vi "test.vi"() -> ()   [LabVIEW 2023]
uses:
  PXI-5441_class/DC Config_class/DC Config.lvclass
  PXI-5441_class/PXI-5441.lvclass
  D:/git/HAL/PXI-5441_class/PXI-5441.lvclass
  D:/git/HAL/FGEN_class/FGEN.lvclass
  D:/git/HAL/Hardware_class/Hardware.lvclass
  D:/git/HAL/PXI-5441_class/DC Config_class/DC Config.lvclass
  D:/git/HAL/PXI-5441_class/IConfigure_interface/IConfigure.lvclass
panel:
  in  "Resource Name":refnum<k15>
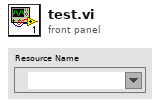
[diagram p1: front panel]
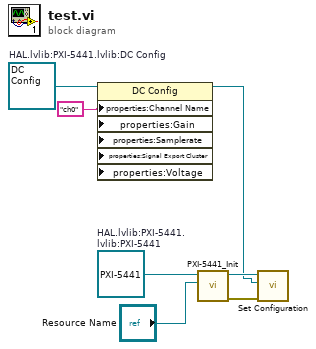
[diagram p0: block diagram]
diagram:
  w7 = refnum<class "PXI-5441.lvclass"> refnum  # HAL.lvlib:PXI-5441.lvlib:PXI-5441
  w3 = refnum<class "DC Config.lvclass"> refnum  # HAL.lvlib:PXI-5441.lvlib:DC Config
  n1 = property class="DC Config" props=["properties:Channel Name", "properties:Gain", "properties:Samplerate", "properties:Signal Export Cluster", "properties:Voltage"](reference=w3, "properties:Channel Name"="ch0" ("Channel Name")) -> (reference out=w2:refnum<class "DC Config.lvclass">)  [unwired: 5 in, 1 out]
  n2 = call "PXI-5441_Init.vi"("Resource Name"="Resource Name", "Object in"=w7) -> ("Error Out"=w5:errorcluster, "object out"=w4:refnum<class "PXI-5441.lvclass">)  [unwired: 8 in]
  n3 = call "Set Configuration.vi"("error in (no error)"=w5, "HAL.lvlib:PXI-5441.lvlib:IConfigure"=w2, "PXI-5441 in"=w4) -> ()  [unwired: 7 in, 2 out]
